vi "Sequence.Test.Unload.Ready.vi"(10 "Data in":T8, 11 "Code":T1={"Ready"=FALSE, "DoubleOrder"=FALSE, "OrderDone"=FALSE, "AllowSingleSlot"=FALSE, "CheckDM"=FALSE, "ThresholdA"=0, "ThresholdB"=0, "Plate"=enum."Wabco", "ImgPath"=path "", "Variant"={"State"=enum."Init", "ImgPath"=path "", "WabcoPlate"="", "WabcoProduct"="", "ClientProduct"="", "ClientPlate"="", "TotalQuantity"=0, "OrderQuantity"=0, "Serial"=0, "Wabco"={"LaserJob"="", "AdditionalTxt"="037", "FactoryCode"="", "RevID"=0, "ForkID"=0, "FailuresLimit"=0, "GlobalCnt"=0, "ScannerProgram"=0, "SerialFormat"=enum."6 dig", "CoordA"={"X"=0.0, "Y"=0.0, "Angle"=0.0}, "CoordB"={"X"=0.0, "Y"=0.0, "Angle"=0.0}, "DMCconfig"=0}, "Client"={"LaserJob"="", "AdditionalTxt"="", "FactoryCode"="037", "RevID"=0, "ForkID"=0, "FailuresLimit"=0, "GlobalCnt"=0, "ScannerProgram"=0, "SerialFormat"=enum."6 dig", "CoordA"={"X"=0.0, "Y"=0.0, "Angle"=0.0}, "CoordB"={"X"=0.0, "Y"=0.0, "Angle"=0.0}, "DMCconfig"=0}}}) -> (2 "OK B":bool, 3 "OK A":bool, 5 "PartialOrder":bool)   [LabVIEW 2016]
uses:
  Sequence.Test.Status.ctl
  Sequence.Slot.StatusData.ctl
  Sequence.Test.Unload.Status.ctl
  Sequence.Prod.StatusData.ctl
  Sequence.Step.Status.ctl
  Sequence.Test.BreakReason.ctl
  Sequence.Code.Sets.ctl
  Sequence.PlateType.ctl
  Logger/Logger.Variant.Sets.ctl
  Station/Station.Changeover.State.vi
  Station/Station.Plate.Properties.ctl
  Sequence.Code.SerialFormat.ctl
  Drivers/V7310/LowLevel/V7310.Job.Sets.ctl
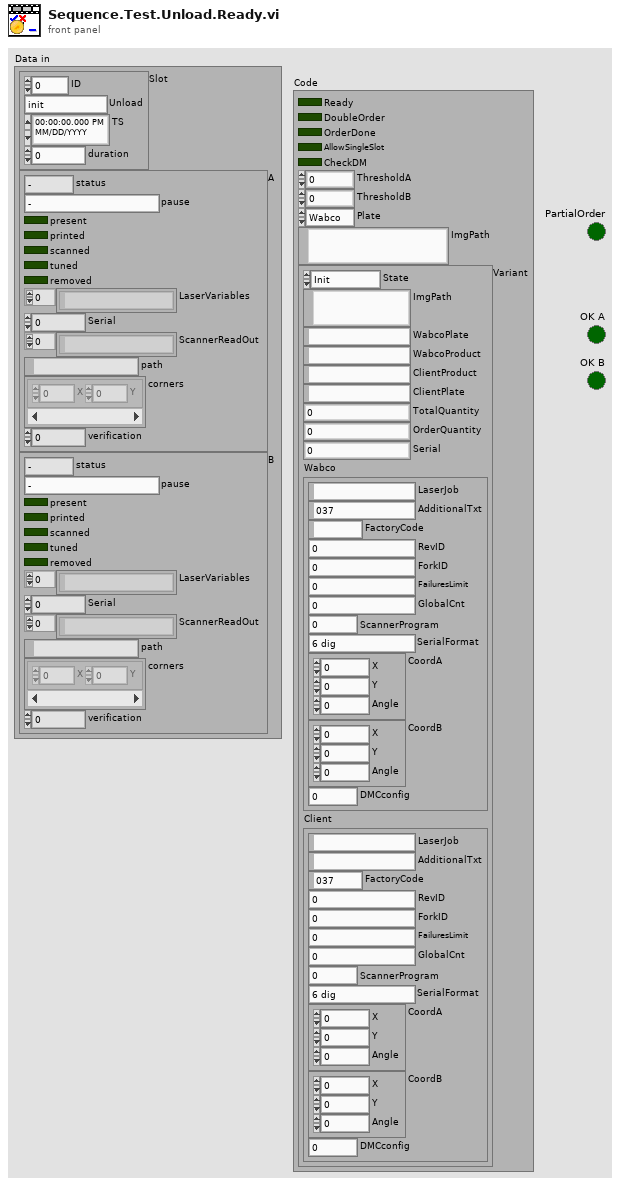
[diagram p1: front panel]
types:
  T1 = typedef "Sequence.Code.Sets.ctl" = cluster{"Ready":bool, "DoubleOrder":bool, "OrderDone":bool, "AllowSingleSlot":bool, "CheckDM":bool, "ThresholdA":u8, "ThresholdB":u8, "Plate":T2, "ImgPath":path, "Variant":T3}
  T2 = typedef "Sequence.PlateType.ctl" = enum16{"Wabco", "Client"}
  T3 = typedef "Logger.Variant.Sets.ctl" = cluster{"State":T4, "ImgPath":path, "WabcoPlate":string, "WabcoProduct":string, "ClientProduct":string, "ClientPlate":string, "TotalQuantity":u16, "OrderQuantity":u16, "Serial":i32, "Wabco":T5, "Client":T5}
  T4 = typedef "Station.Changeover.State.vi" = enum16{"Init", "Scaning", "NOK", "Wait for ack", "Ready"}
  T5 = typedef "Station.Plate.Properties.ctl" = cluster{"LaserJob":string, "AdditionalTxt":string, "FactoryCode":string, "RevID":u8, "ForkID":u8, "FailuresLimit":u16, "GlobalCnt":i32, "ScannerProgram":u8, "SerialFormat":T6, "CoordA":T7, "CoordB":T7, "DMCconfig":i32}
  T6 = typedef "Sequence.Code.SerialFormat.ctl" = enum8{"", "6 dig", "7 dig"}
  T7 = typedef "V7310.Job.Sets.ctl" = cluster{"X":dbl, "Y":dbl, "Angle":dbl}
  T8 = typedef "Sequence.Test.Status.ctl" = cluster{"Slot":T9, "A":T11, "B":T11}
  T9 = typedef "Sequence.Slot.StatusData.ctl" = cluster{"ID":i32, "Unload":T10, "TS":timestamp, "duration":u32}
  T10 = typedef "Sequence.Test.Unload.Status.ctl" = enum16{"init", "check NOK", "check OK", "wait on NOK", "wait on OK", "wait on Unload", "done"}
  T11 = typedef "Sequence.Prod.StatusData.ctl" = cluster{"status":T12, "pause":T13, "present":bool, "printed":bool, "scanned":bool, "tuned":bool, "removed":bool, "LaserVariables":string[], "Serial":i32, "ScannerReadOut":string[], "path":path, "corners":cluster{"X":i32, "Y":i32}[], "verification":u8}
  T12 = typedef "Sequence.Step.Status.ctl" = enum16{"-", "Pending", "Running", "Skipped", "Passed", "Failed", "Done", "Error", "Aborted", "Stopped"}
  T13 = typedef "Sequence.Test.BreakReason.ctl" = enum16{"-", "NOK container", "OK container", "Rev empty", "Rev missing", "Rev wrong", "Fork missing", "Fork wrong", "NOK limit", "Unload failure", "Single slot", "Part done", "Err: Prod move work", "Err: Prod move home", "Err: Prod lift work", "Err: Prod lift home", "Err: Prod Arm Work", "Err: Prod Arm NOK", "Err: Prod Arm OK", "Err: Prod NOK suck", "Err: Prod NOK drop", "Err: Prod OK missing", "Err: Prod OK suck", "Err: Prod OK drop"}
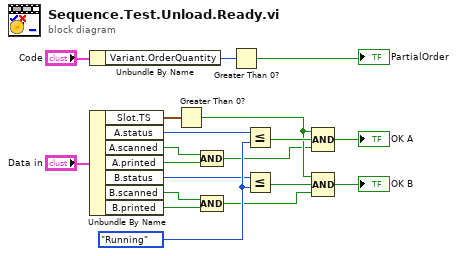
[diagram p0: block diagram]
diagram:
  w19 = Sequence.Step.Status."Running" ("y")
  n1 = Unbundle By Name("Code") -> ("Variant.OrderQuantity"=w8:u16)
  n2 = Unbundle By Name("Data in") -> ("Slot.TS"=w4:timestamp, "A.status"=w18:T12, "A.scanned"=w12:bool, "A.printed"=w11:bool, "B.status"=w17:T12, "B.scanned"=w10:bool, "B.printed"=w9:bool)
  n3 = Greater Than 0?(x=w4) -> (x > 0?=w3:bool)
  n4 = Compound Arithmetic op=AND(w12, w11) -> (w2:bool)
  n5 = Compound Arithmetic op=AND(w10, w9) -> (w1:bool)
  n6 = Greater Than 0?(x=w8) -> (x > 0?=→"PartialOrder":bool)
  n7 = Less Or Equal?(x=w18, y=w19) -> (x <= y?=w14:bool)
  n8 = Less Or Equal?(x=w17, y=w19) -> (x <= y?=w5:bool)
  n9 = Compound Arithmetic op=AND(w3, w14, w2) -> (→"OK A":bool)
  n10 = Compound Arithmetic op=AND(w3, w5, w1) -> (→"OK B":bool)
